vi "Parse GGA Sentence.vi"(7 "date override":timestamp format="%<%x>T", 8 "error in (no error)":errorcluster, 11 "GGA sentence":string) -> (0 "error out":errorcluster, 3 "GGA data":T1 {"fix quality"."quality" items=["Invalid", "GPS Fix", "DGPS Fix", "PPS Fix", "Real Time Kinematic", "Float RTK", "Estimated", "Manual Input Mode", "Simulation Mode"]; "time of fix"."time" format="%^<%.3X\n%x>T"})   [LabVIEW 2009]
doc: "Returns data contained in an NMEA sentence. You must manually select the polymorphic instance to use."
uses:
  typedefs/GGA Data.ctl
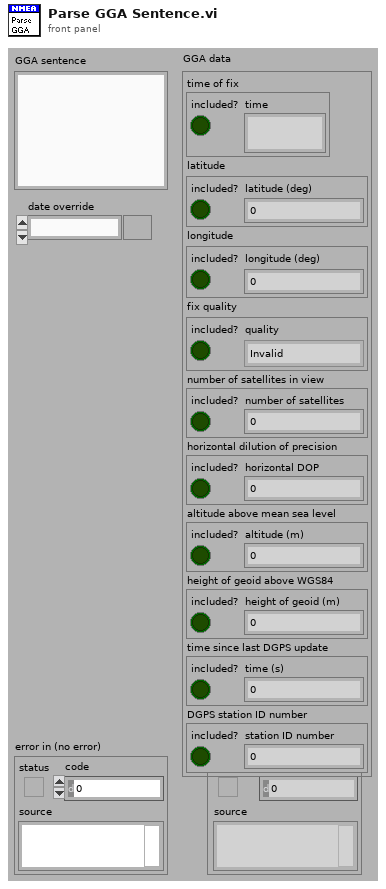
[diagram p1: front panel]
types:
  T1 = typedef "GGA Data.ctl" = cluster{"time of fix":cluster{"included?":bool, "time":timestamp}, "latitude":cluster{"included?":bool, "latitude (deg)":dbl}, "longitude":cluster{"included?":bool, "longitude (deg)":dbl}, "fix quality":cluster{"included?":bool, "quality":u16}, "number of satellites in view":cluster{"included?":bool, "number of satellites":i8}, "horizontal dilution of precision":cluster{"included?":bool, "horizontal DOP":dbl}, "altitude above mean sea level":cluster{"included?":bool, "altitude (m)":dbl}, "height of geoid above WGS84":cluster{"included?":bool, "height of geoid (m)":dbl}, "time since last DGPS update":cluster{"included?":bool, "time (s)":dbl}, "DGPS station ID number":cluster{"included?":bool, "station ID number":dbl}}
  T2 = cluster{"Valid?":bool, "Number of Satellites":i8}
  T3 = typedef "LVDateTimeRec.ctl" = cluster{"fractional second":dbl, "second":i32, "minute":i32, "hour":i32, "day of month":i32, "month":i32, "year":i32, "day of week":i32, "day of year":i32, "DST":i32}
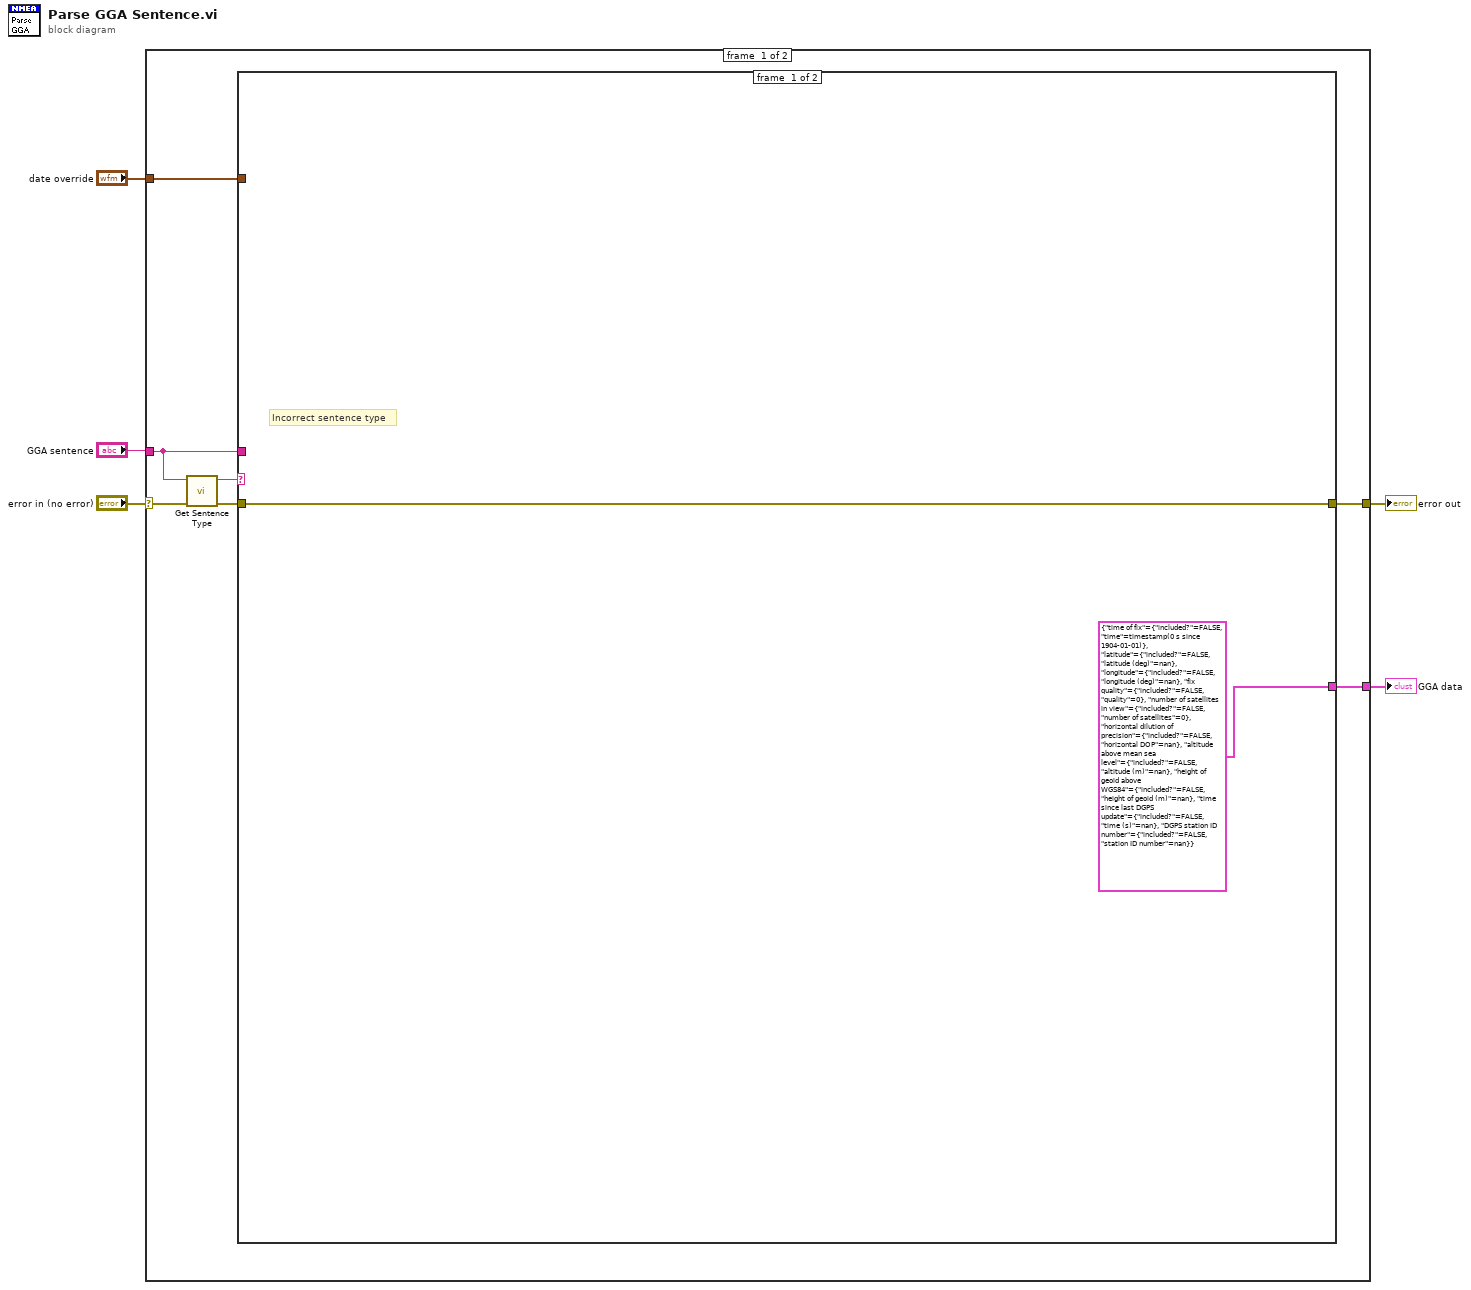
[diagram p0: block diagram]
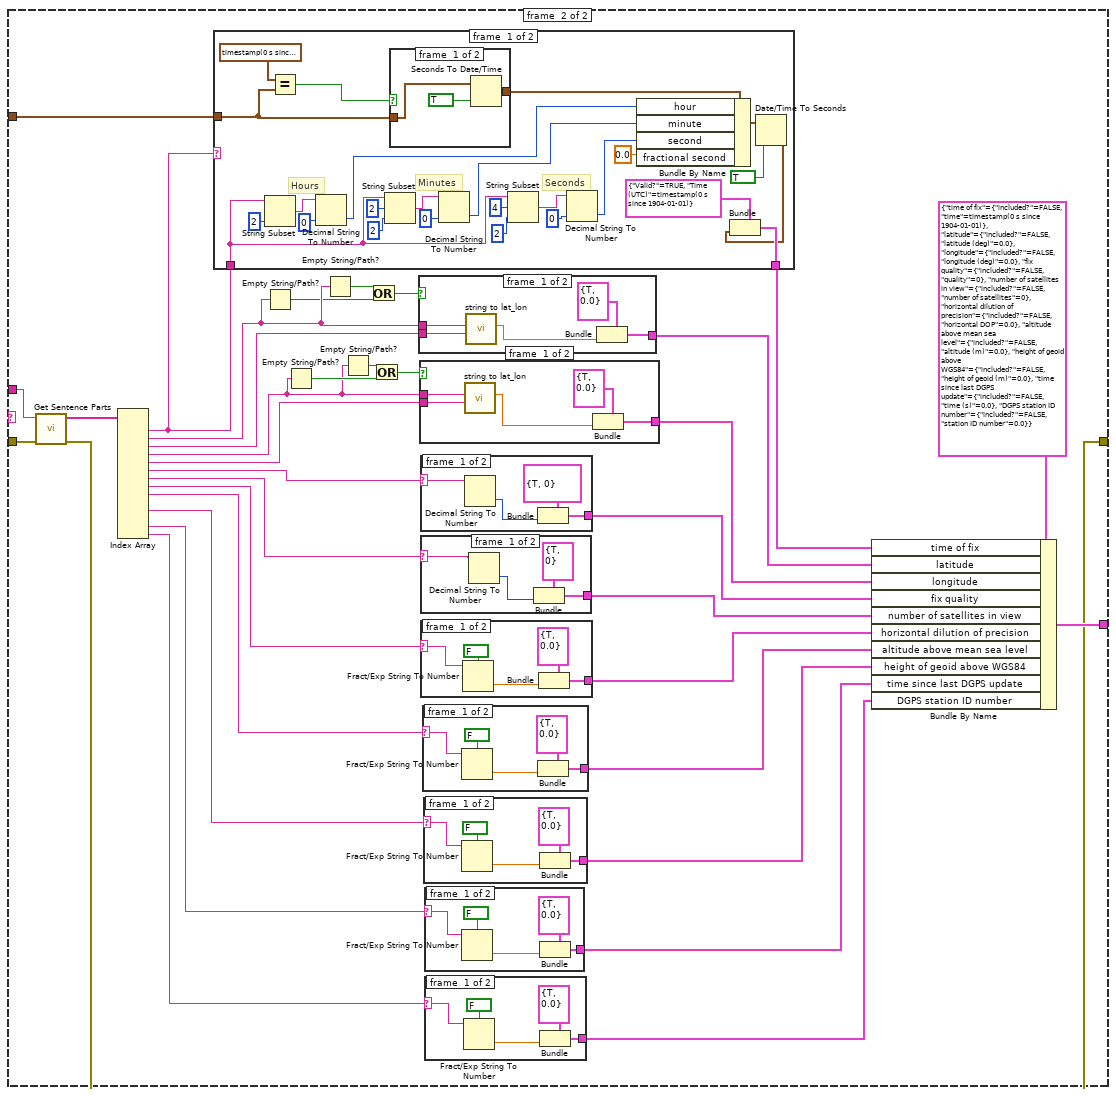
[diagram p2: hidden frame]
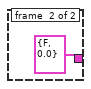
[diagram p3: hidden frame]
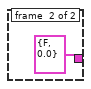
[diagram p4: hidden frame]
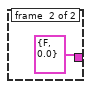
[diagram p5: hidden frame]
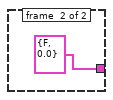
[diagram p6: hidden frame]
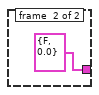
[diagram p7: hidden frame]
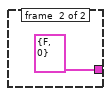
[diagram p8: hidden frame]
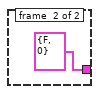
[diagram p9: hidden frame]
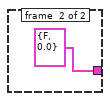
[diagram p10: hidden frame]
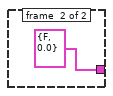
[diagram p11: hidden frame]
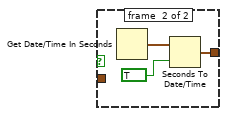
[diagram p12: hidden frame]
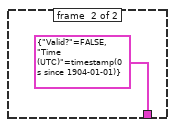
[diagram p13: hidden frame]
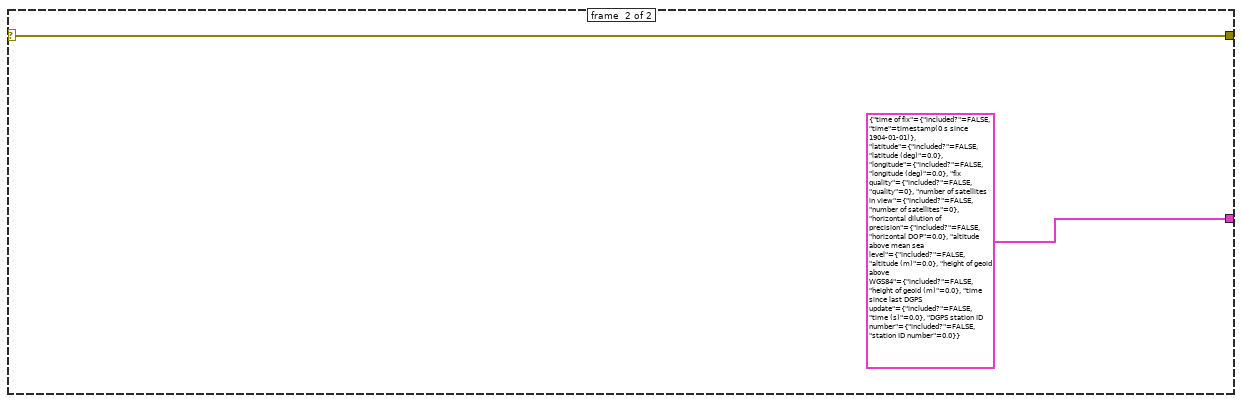
[diagram p14: hidden frame]
diagram:
  n1 = case shown="No Error" "error in (no error)" {
    selector: "error in (no error)" -> [w9 w135]
    tunnel: [w10 w135] -> w3
    tunnel: [w12 T1 {"time of fix"={"included?"=FALSE, "time"=timestamp(0 s since 1904-01-01)}, "latitude"={"included?"=FALSE, "latitude (deg)"=0.0}, "longitude"={"included?"=FALSE, "longitude (deg)"=0.0}, "fix quality"={"included?"=FALSE, "quality"=0}, "number of satellites in view"={"included?"=FALSE, "number of satellites"=0}, "horizontal dilution of precision"={"included?"=FALSE, "horizontal DOP"=0.0}, "altitude above mean sea level"={"included?"=FALSE, "altitude (m)"=0.0}, "height of geoid above WGS84"={"included?"=FALSE, "height of geoid (m)"=0.0}, "time since last DGPS update"={"included?"=FALSE, "time (s)"=0.0}, "DGPS station ID number"={"included?"=FALSE, "station ID number"=0.0}} ("GGA Data")] -> w2
    tunnel: "GGA sentence" -> [w7 _]
    tunnel: "date override" -> [w11 _]
    frame #0 {
      n2 = call "Get Sentence Type.vi"("error in (no error)"=w9, "sentence"=w7) -> ("error out"=w8:errorcluster, "sentence type"=w6:string)  [unwired: 1 in, 7 out]
      n3 = case shown="\"GPGGA\"" w6 {
        tunnel: [T1 {"time of fix"={"included?"=FALSE, "time"=timestamp(0 s since 1904-01-01)}, "latitude"={"included?"=FALSE, "latitude (deg)"=nan}, "longitude"={"included?"=FALSE, "longitude (deg)"=nan}, "fix quality"={"included?"=FALSE, "quality"=0}, "number of satellites in view"={"included?"=FALSE, "number of satellites"=0}, "horizontal dilution of precision"={"included?"=FALSE, "horizontal DOP"=nan}, "altitude above mean sea level"={"included?"=FALSE, "altitude (m)"=nan}, "height of geoid above WGS84"={"included?"=FALSE, "height of geoid (m)"=nan}, "time since last DGPS update"={"included?"=FALSE, "time (s)"=nan}, "DGPS station ID number"={"included?"=FALSE, "station ID number"=nan}} ("GGA Data") w49] -> w12
        tunnel: w7 -> [_ w16]
        tunnel: w8 -> [w13 w48]
        tunnel: w11 -> [_ w47]
        tunnel: [w13 w30] -> w10
        frame #0 {
          # "Incorrect sentence type"
        }
        frame #1 {
          n4 = call "Get Sentence Parts.vi"("error in (no error)"=w48, "sentence"=w16) -> ("error out"=w30:errorcluster, "sentence data"=w15:string[])  [unwired: 1 in, 7 out]
          n5 = Index Array(array=w15) -> (element #1=w24:string, element #2=w42:string, element #3=w46:string, element #4=w38:string, element #5=w45:string, element #6=w23:string, element #7=w22:string, element #8=w21:string, element #9=w20:string, element #11=w19:string, element #13=w18:string, element #14=w17:string)  [unwired: 14 in, 2 out]
          n6 = case shown="\"False\", Default" w24 {
            tunnel: w47 -> [w124 _]
            tunnel: [w108 cluster{"Valid?":bool, "Time (UTC)":timestamp} {"Valid?"=FALSE, "Time (UTC)"=timestamp(0 s since 1904-01-01)} ("Time of Fix")] -> w36
            tunnel: w24 -> [w109 _]
            frame #0 {
              # "Seconds"
              # "Minutes"
              # "Hours"
              n7 = String Subset(string=w109, length (rest)=2 ("length (rest)")) -> (substring=w116:string)  [unwired: 1 out]
              n8 = Equal?(x=timestamp(0 s since 1904-01-01), y=w124) -> (x = y?=w126:bool)
              n9 = Decimal String To Number(string=w116, default (0L)=0 ("default (0 DBL)")) -> (number=w110:i32)  [unwired: 2 out]
              n10 = String Subset(string=w109, offset (0)=2, length (rest)=2 ("length (rest)")) -> (substring=w117:string)
              n11 = case shown="True" w126 {
                tunnel: w124 -> [w129 _]
                tunnel: [w128 w131] -> w114
                frame #0 {
                  n12 = Seconds To Date/Time(time stamp (now)=w129, to UTC (F)=TRUE) -> (date time rec=w128:T3)
                }
                frame #1 {
                  n13 = Get Date/Time In Seconds() -> (seconds since 1Jan1904=w132:timestamp)
                  n14 = Seconds To Date/Time(time stamp (now)=w132, to UTC (F)=TRUE) -> (date time rec=w131:T3)
                }
              }
              n15 = Decimal String To Number(string=w117, default (0L)=0 ("default (0 DBL)")) -> (number=w111:i32)  [unwired: 2 out]
              n16 = String Subset(string=w109, offset (0)=4, length (rest)=2 ("length (rest)")) -> (substring=w120:string)
              n17 = Decimal String To Number(string=w120, default (0L)=0 ("default (0 DBL)")) -> (number=w112:i32)  [unwired: 2 out]
              n18 = Bundle By Name(cluster=w114, "hour"=w110, "minute"=w111, "second"=w112, "fractional second"=0.0) -> (w113:T3)
              n19 = Date/Time To Seconds(1:TRUE, 2:w113) -> (0:w106:timestamp)
              n20 = Bundle(cluster=cluster{"Valid?":bool, "Time (UTC)":timestamp} {"Valid?"=TRUE, "Time (UTC)"=timestamp(0 s since 1904-01-01)} ("Time of Fix"), "Time (UTC)"=w106) -> (w108:cluster{"Valid?":bool, "Time (UTC)":timestamp})  [unwired: 1 out]
            }
            frame #1 {
            }
          }
          n21 = Empty String/Path?(string/path=w42) -> (empty?=w41:bool)
          n22 = Empty String/Path?(string/path=w38) -> (empty?=w40:bool)
          n23 = Empty String/Path?(string/path=w42) -> (empty?=w43:bool)
          n24 = Empty String/Path?(string/path=w38) -> (empty?=w39:bool)
          n25 = Or(x=w43, y=w41) -> (x .or. y?=w44:bool)
          n26 = Or(x=w39, y=w40) -> (x .or. y?=w37:bool)
          n27 = case shown="False" w44 {
            tunnel: [w98 cluster{"Valid?":bool, "Latitude (Deg)":dbl} {"Valid?"=FALSE, "Latitude (Deg)"=0.0} ("Latitude")] -> w33
            tunnel: w42 -> [w100 _]
            tunnel: w46 -> [w99 _]
            frame #0 {
              n28 = call "string to lat_lon.vi"("direction string"=w99, "numeric string for lat/lon"=w100) -> ("composite value"=w96:dbl)  [unwired: 1 in, 8 out]
              n29 = Bundle(cluster=cluster{"Valid?":bool, "Latitude (Deg)":dbl} {"Valid?"=TRUE, "Latitude (Deg)"=0.0} ("Latitude"), "Latitude (Deg)"=w96) -> (w98:cluster{"Valid?":bool, "Latitude (Deg)":dbl})  [unwired: 1 out]
            }
            frame #1 {
            }
          }
          n30 = case shown="False" w37 {
            tunnel: w45 -> [w94 _]
            tunnel: w38 -> [w93 _]
            tunnel: [w90 cluster{"Valid?":bool, "Longitude (Deg)":dbl} {"Valid?"=FALSE, "Longitude (Deg)"=0.0} ("Longitude")] -> w31
            frame #0 {
              n31 = call "string to lat_lon.vi"("direction string"=w94, "numeric string for lat/lon"=w93) -> ("composite value"=w92:dbl)  [unwired: 1 in, 8 out]
              n32 = Bundle(cluster=cluster{"Valid?":bool, "Longitude (Deg)":dbl} {"Valid?"=TRUE, "Longitude (Deg)"=0.0} ("Longitude"), "Longitude (Deg)"=w92) -> (w90:cluster{"Valid?":bool, "Longitude (Deg)":dbl})  [unwired: 1 out]
            }
            frame #1 {
            }
          }
          n33 = case shown="\"False\", Default" w23 {
            selector: w23 -> [w85 _]
            tunnel: [w86 cluster{"Valid?":bool, "Fix Quality":u16} {"Valid?"=FALSE, "Fix Quality"=0} ("Fix Quality")] -> w35
            frame #0 {
              n34 = Decimal String To Number(string=w85) -> (number=w87:i32)  [unwired: 3 out]
              n35 = Bundle(cluster=cluster{"Valid?":bool, "Fix Quality":u16} {"Valid?"=TRUE, "Fix Quality"=0} ("Fix Quality"), "Fix Quality"=w87) -> (w86:cluster{"Valid?":bool, "Fix Quality":u16})  [unwired: 1 out]
            }
            frame #1 {
            }
          }
          n36 = case shown="\"False\", Default" w22 {
            selector: w22 -> [w80 _]
            tunnel: [w81 T2 {"Valid?"=FALSE, "Number of Satellites"=0} ("Number of Satellites Being Tracked")] -> w34
            frame #0 {
              n37 = Decimal String To Number(string=w80) -> (number=w83:i32)  [unwired: 3 out]
              n38 = Bundle(cluster=T2 {"Valid?"=TRUE, "Number of Satellites"=0} ("Number of Satellites Being Tracked"), "Number of Satellites"=w83) -> (w81:T2)  [unwired: 1 out]
            }
            frame #1 {
            }
          }
          n39 = case shown="\"False\", Default" w21 {
            selector: w21 -> [w75 _]
            tunnel: [w76 cluster{"Valid?":bool, "Horizontal DOP":dbl} {"Valid?"=FALSE, "Horizontal DOP"=0.0} ("Horizontal Dilution of Precision")] -> w29
            frame #0 {
              n40 = Fract/Exp String To Number(use system decimal point (T)=FALSE, string=w75) -> (number=w77:dbl)  [unwired: 3 out]
              n41 = Bundle(cluster=cluster{"Valid?":bool, "Horizontal DOP":dbl} {"Valid?"=TRUE, "Horizontal DOP"=0.0} ("Horizontal Dilution of Precision"), "Horizontal DOP"=w77) -> (w76:cluster{"Valid?":bool, "Horizontal DOP":dbl})  [unwired: 1 out]
            }
            frame #1 {
            }
          }
          n42 = case shown="\"False\", Default" w20 {
            selector: w20 -> [w69 _]
            tunnel: [w70 cluster{"Valid?":bool, "Horizontal DOP":dbl} {"Valid?"=FALSE, "Horizontal DOP"=0.0} ("Horizontal Dilution of Precision")] -> w28
            frame #0 {
              n43 = Fract/Exp String To Number(use system decimal point (T)=FALSE, string=w69) -> (number=w71:dbl)  [unwired: 3 out]
              n44 = Bundle(cluster=cluster{"Valid?":bool, "Horizontal DOP":dbl} {"Valid?"=TRUE, "Horizontal DOP"=0.0} ("Horizontal Dilution of Precision"), "Horizontal DOP"=w71) -> (w70:cluster{"Valid?":bool, "Horizontal DOP":dbl})  [unwired: 1 out]
            }
            frame #1 {
            }
          }
          n45 = case shown="\"False\", Default" w19 {
            selector: w19 -> [w63 _]
            tunnel: [w64 cluster{"Valid?":bool, "Horizontal DOP":dbl} {"Valid?"=FALSE, "Horizontal DOP"=0.0} ("Horizontal Dilution of Precision")] -> w27
            frame #0 {
              n46 = Fract/Exp String To Number(use system decimal point (T)=FALSE, string=w63) -> (number=w65:dbl)  [unwired: 3 out]
              n47 = Bundle(cluster=cluster{"Valid?":bool, "Horizontal DOP":dbl} {"Valid?"=TRUE, "Horizontal DOP"=0.0} ("Horizontal Dilution of Precision"), "Horizontal DOP"=w65) -> (w64:cluster{"Valid?":bool, "Horizontal DOP":dbl})  [unwired: 1 out]
            }
            frame #1 {
            }
          }
          n48 = case shown="\"False\", Default" w18 {
            selector: w18 -> [w57 _]
            tunnel: [w58 cluster{"Valid?":bool, "Horizontal DOP":dbl} {"Valid?"=FALSE, "Horizontal DOP"=0.0} ("Horizontal Dilution of Precision")] -> w26
            frame #0 {
              n49 = Fract/Exp String To Number(use system decimal point (T)=FALSE, string=w57) -> (number=w59:dbl)  [unwired: 3 out]
              n50 = Bundle(cluster=cluster{"Valid?":bool, "Horizontal DOP":dbl} {"Valid?"=TRUE, "Horizontal DOP"=0.0} ("Horizontal Dilution of Precision"), "Horizontal DOP"=w59) -> (w58:cluster{"Valid?":bool, "Horizontal DOP":dbl})  [unwired: 1 out]
            }
            frame #1 {
            }
          }
          n51 = case shown="\"False\", Default" w17 {
            selector: w17 -> [w51 _]
            tunnel: [w52 cluster{"Valid?":bool, "Horizontal DOP":dbl} {"Valid?"=FALSE, "Horizontal DOP"=0.0} ("Horizontal Dilution of Precision")] -> w25
            frame #0 {
              n52 = Fract/Exp String To Number(use system decimal point (T)=FALSE, string=w51) -> (number=w53:dbl)  [unwired: 3 out]
              n53 = Bundle(cluster=cluster{"Valid?":bool, "Horizontal DOP":dbl} {"Valid?"=TRUE, "Horizontal DOP"=0.0} ("Horizontal Dilution of Precision"), "Horizontal DOP"=w53) -> (w52:cluster{"Valid?":bool, "Horizontal DOP":dbl})  [unwired: 1 out]
            }
            frame #1 {
            }
          }
          n54 = Bundle By Name(cluster=T1 {"time of fix"={"included?"=FALSE, "time"=timestamp(0 s since 1904-01-01)}, "latitude"={"included?"=FALSE, "latitude (deg)"=0.0}, "longitude"={"included?"=FALSE, "longitude (deg)"=0.0}, "fix quality"={"included?"=FALSE, "quality"=0}, "number of satellites in view"={"included?"=FALSE, "number of satellites"=0}, "horizontal dilution of precision"={"included?"=FALSE, "horizontal DOP"=0.0}, "altitude above mean sea level"={"included?"=FALSE, "altitude (m)"=0.0}, "height of geoid above WGS84"={"included?"=FALSE, "height of geoid (m)"=0.0}, "time since last DGPS update"={"included?"=FALSE, "time (s)"=0.0}, "DGPS station ID number"={"included?"=FALSE, "station ID number"=0.0}} ("GGA Data"), "time of fix"=w36, "latitude"=w33, "longitude"=w31, "fix quality"=w35, "number of satellites in view"=w34, "horizontal dilution of precision"=w29, "altitude above mean sea level"=w28, "height of geoid above WGS84"=w27, "time since last DGPS update"=w26, "DGPS station ID number"=w25) -> (w49:T1)
        }
      }
    }
    frame #1 {
    }
  }
  "error out" <- w3
  "GGA data" <- w2
